vi "to string array.vi"(8 "error in (no error)":errorcluster, 11 "Sequencer Module configuration in":refnum<class "Sequencer Module configuration.lvclass">) -> (0 "error out":errorcluster, 1 "Array":string[][](array[string]), 2 "version":string, 3 "Sequencer Module configuration out":refnum<class "Sequencer Module configuration.lvclass">)   [LabVIEW 2015, in "Sequencer Module configuration.lvclass"]
uses:
  Sequencer Module configuration.lvclass
  Sequencer Module configuration.lvclass/Sequencer Module configuration.ctl
  Read Lines.vi
  classes/Sequence/Config/Sequence Config.lvclass
  <vilib>/NI/Tag Bus/tag/tag descriptor.lvclass
  <vilib>/NI/Tag Bus Module Framework/channel/TBM channel.lvclass
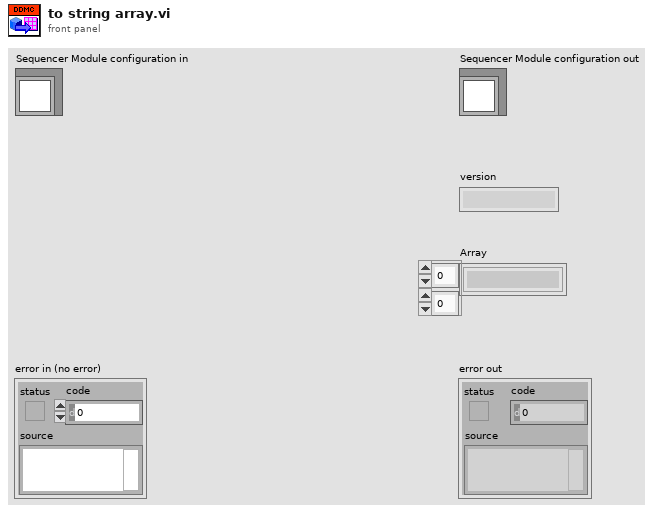
[diagram p1: front panel]
types:
  T1 = typedef "Sequencer Module configuration.lvclass/Line.ctl" = cluster{"Sequence":refnum<class "Sequence Config.lvclass">}
  T2 = typedef "TBM channel.lvclass/channel classification.ctl" = enum16{"input data", "output data", "processing parameter", "processing result"}
  T3 = typedef "tag bus.lvlib/tag descriptor.lvclass/Data Type.ctl" = enum16{"Double", "Single", "I64", "I32", "I16", "I8", "U64", "U32", "U16", "U8", "Boolean", "String", "Array of Double", "Array of Single", "Array of I64", "Array of I32", "Array of I16", "Array of I8", "Array of U64", "Array of U32", "Array of U16", "Array of U8", "Array of Boolean", "Array of String"}
  T4 = typedef "Sequencer Module configuration.lvclass/permissions.ctl" = enum32{"Read from HW", "Write to HW"}
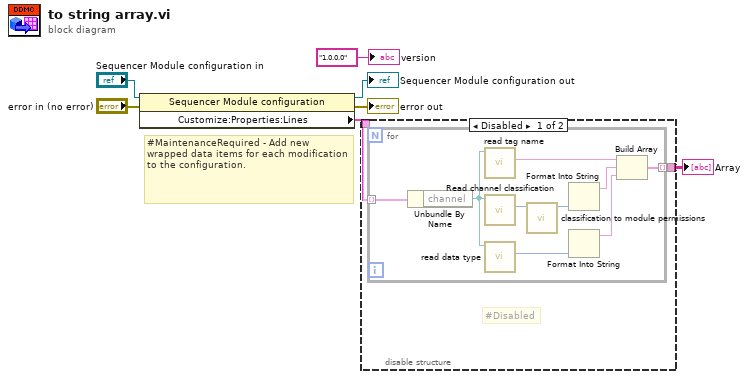
[diagram p0: block diagram]
diagram:
  # "#MaintenanceRequired - Add new wrapped data items for each modification to the configuration."
  n1 = property class="Sequencer Module configuration"(reference="Sequencer Module configuration in", error in="error in (no error)") -> (reference out=→"Sequencer Module configuration out":refnum<class "Sequencer Module configuration.lvclass">, error out=→"error out":errorcluster, "Customize:Properties:Lines"=w4:T1[])
  n2 = disable-structure shown="Disabled" {
    disable-tunnel: w4 -> [w9 _]
    disable-tunnel: [w8 _] -> w1
    frame Disabled {
      # "#Disabled"
      n3 = for {
        tunnel: w9 -> [w18] mode=indexing
        tunnel: [w10] -> w8 mode=indexing
        n4 = Unbundle By Name(w18) -> ("channel"=w13:refnum<class "TBM channel.lvclass">)
        n5 = call <vilib>:"read tag name.vi"("system tag in"=w13) -> ("name"=w17:string)  [unwired: 8 in, 2 out]
        n6 = call <vilib>:"Read channel classification.vi"("channel in"=w13) -> ("channel classification"=w16:T2)  [unwired: 8 in, 2 out]
        n7 = call <vilib>:"read data type.vi"("system tag in"=w13) -> ("data type"=w12:T3)  [unwired: 8 in, 2 out]
        n8 = call "classification to module permissions.vi"("channel classification"=w16) -> ("permissions"=w15:T4)  [unwired: 10 in]
        n9 = Format Into String(w15) -> (resulting string=w14:string)  [unwired: 3 in, 1 out]
        n10 = Format Into String(w12) -> (resulting string=w11:string)  [unwired: 3 in, 1 out]
        n11 = Build Array(w17, w14, w11) -> (w10:string[])
      }
    }
    frame Enabled {
    }
  }
  "Array" <- w1
  "version" <- "1.0.0.0" ("version")
